vi "SVXMPL_Noisy Sine Wave (simulated).vi"(6 "sampling info":cluster{"Fs":dbl, "#s":dbl} {"#s" format="%.2f"; "Fs" format="%.2f"}, 8 "error in (no error)":errorcluster, 9 "channel info":T1={"sensor sensitivity [mV/EU]"=1000.0, "engineering units"=enum."V", "dB reference [EU]"=1.0, "custom label"="EU", "weighting filter"=enum."Linear", "pregain [dB]"=0.0} {"pregain [dB]" format="%.2f"; "dB reference [EU]" format="%.1e"; "sensor sensitivity [mV/EU]" format="%.2f"}, 10 "noise":dbl=0.01 format="%.2f", 11 "frequency":dbl=10.0 format="%.2p") -> (0 "error out":errorcluster, 2 "unit label":string, 3 "noisy sine wave":waveform(dbl))   [LabVIEW 2017]
uses:
  <vilib>/addons/Sound and Vibration/svt_Calibration/SVL Scale Voltage to EU (1 Ch).vi
  <vilib>/addons/_NISVFA/_Shared subVIs/Common/svc_Set SV Channel Info.vi
  <vilib>/addons/_NISVFA/_Shared subVIs/Common/svc_Set SV Channel Info (variant).vi
  <vilib>/addons/_NISVFA/_Shared subVIs/Common/SVL Set dB Reference (variant).vi
  <vilib>/addons/_NISVFA/_Shared subVIs/Common/svc_Caller VI Returned in Error Source.vi
  <vilib>/addons/_NISVFA/_Shared subVIs/Common/svc_Engineering Units to Unit Label.vi
  <vilib>/addons/_NISVFA/_Shared subVIs/Common/svc_Set dB ref if Pascal.vi
  <vilib>/addons/_NISVFA/_Shared subVIs/Common/svc_Compute Scale Factor to Convert C to EU.vi
  <vilib>/addons/_NISVFA/_Shared subVIs/Common/svc_Compute Scale Factor to Convert V to EU.vi
  <vilib>/measure/NI_MABase.lvlib
  <vilib>/addons/Sound and Vibration/svt_Calibration/SoundVib_Calibration.lvlib
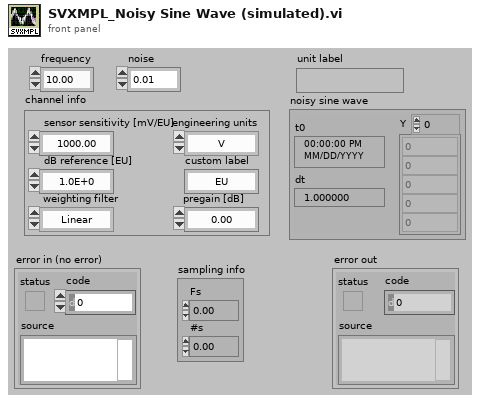
[diagram p1: front panel]
types:
  T1 = cluster{"sensor sensitivity [mV/EU]":dbl, "engineering units":enum16{"custom...", "V", "Pa", "g", "m/s^2", "m/s", "m", "in/s^2", "in/s", "in"}, "dB reference [EU]":dbl, "custom label":string, "weighting filter":enum16{"Linear", "A-weighting", "B-weighting", "C-weighting"}, "pregain [dB]":dbl}
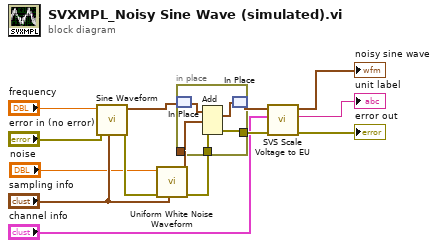
[diagram p0: block diagram]
diagram:
  n1 = call <vilib>:"Sine Waveform.vi"("sampling info"="sampling info", "error in (no error)"="error in (no error)", "frequency"="frequency") -> ("error out"=w12:errorcluster, "signal out"=w9:waveform(dbl))  [unwired: 7 in]
  n2 = call <vilib>:"Uniform White Noise Waveform.vi"("sampling info"="sampling info", "error in (no error)"=w12, "amplitude"="noise") -> ("error out"=w13:errorcluster, "signal out"=w10:waveform(dbl))  [unwired: 7 in]
  n3 = in-place {
    in-place-border: w13 -> [w19]
    in-place-border: w10 -> [w18]
    in-place-border: [w15] -> w4
    n4 = in-place-match #1(w9) -> (w17:waveform(dbl))
    n5 = Add ("Add Waveforms.vi")(1:w18, 2:w17, 4:w19) -> (0:w16:waveform(dbl), 3:w15:errorcluster)
    n6 = in-place-match #1(w16) -> (w6:waveform(dbl))
  }
  n7 = call-poly <vilib>:"SVS Scale Voltage to EU.vi"("error in (no error)"=w4, "channel info"="channel info", "signal [V]"=w6) -> ("error out"=→"error out":errorcluster, "unit label"=→"unit label":string, "scaled signal [EU]"=→"noisy sine wave":waveform(dbl))  [unwired: 6 in]
